vi "DRC Get Data.vi"(2 "Point #":i32, 3 "Command String":string, 4 "Instrument Address":refnum<visa-resource-name>) -> (0 "Stop":bool, 1 "Output":dbl[](array[numeric]) format="%.2f")   [LabVIEW 2020]
doc: "This VI reads the sample output of the Lakeshore DRC 93C or 82C temperature controller. The output is an array consisting of the single reading. The input is the numeric GPIB address.\nScott Hannahs, F. Bitter National Magnet Lab, 1993"
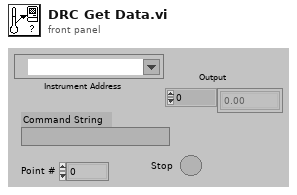
[diagram p1: front panel]
types:
  T1 = cluster{"Instrument":string, "ID Test String":string, "Terminator Character":string, u32, bool}
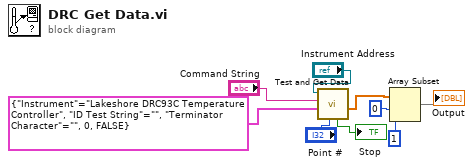
[diagram p0: block diagram]
diagram:
  n1 = call "Test and Get Data.vi"("Point #"="Point #", "Instrument Info"=T1 {"Instrument"="Lakeshore DRC93C Temperature Controller", "ID Test String"="", "Terminator Character"="", 0, FALSE}, "Command String"="Command String", "VISA Sesson"="Instrument Address") -> ("Measurement"=w6:dbl[], "Stop"=→"Stop":bool)  [unwired: 2 in, 3 out]
  n2 = Array Subset(array=w6, index=0, length=1) -> (→"Output":dbl[])
